vi "{TMPL} MAIN - App.vi"() -> ()   [LabVIEW 2015, in "TLB` Template.lvlib" / "{TMPL} TLB`.lvclass"]
uses:
  {TMPL} TLB`.lvclass
  Application Components/Trigger API/System Trigger.ctl
  State Machine/State.ctl
  Core Components/Error Handler/TLB` Error Handler.lvclass
  Application Components/Configuration/{TMPL} Station Configuration.lvclass
  {TMPL} TLB`.lvclass/{TMPL} TLB`.ctl
  <vilib>/Utility/error.llb/Error Cluster From Error Code.vi
  <vilib>/ErrorRing/Error Ring.xnode
  Application Components/Trigger API/{TMPL} Trigger API.lvlib
  TLB` Template.lvlib
  Core Components/Actions/Actions.lvlib
  Core Components/Dependencies/TLB`_Dependencies.lvlib
panel:
  out "error out":errorcluster
  out "State":string
  out "Status":string
  # "TLB` Template"
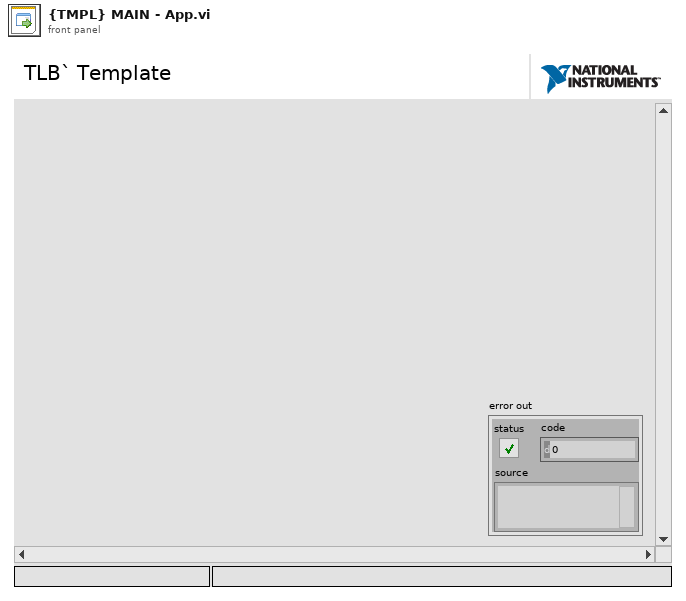
[diagram p1: front panel]
types:
  T1 = typedef "TLB` Template.lvlib/{TMPL} TLB`.lvclass/State.ctl" = enum16{"<Startup>", "Idle", "<Shutdown>", "<Error>"}
  T2 = enum16{"Close Display", "Clear References", "Close Error Handler"}
  T3 = enum16{"Clear SR", "Set Display", "Set Shifter", "Initialize Events", "Init Q"}
  T4 = typedef "TLB` Template.lvlib/{TMPL} Trigger API.lvlib/System Trigger.ctl" = enum16{"<None>", "Connect", "Start Acquisition", "Stop Acquisition", "Disconnect", "<Return to Safe State Actions>", "<Cache User Parameters>", "<Close Application>", "<Error>"}
  T5 = refnum<class "{TMPL} Station Configuration.lvclass">
  T6 = typedef "TLB` Template.lvlib/_UI CORE Event References.ctl" = cluster{"Exit Event":refnum<user-event>, "State Indicator":refnum<user-event>, "Status Indicator":refnum<user-event>}
  T7 = typedef "TLB` Template.lvlib/_UI APP Event References.ctl" = cluster{"Exit Event":refnum<user-event>}
  T8 = enum32{"Invalid", "Standard", "Closed", "Hidden", "Minimized", "Maximized"}
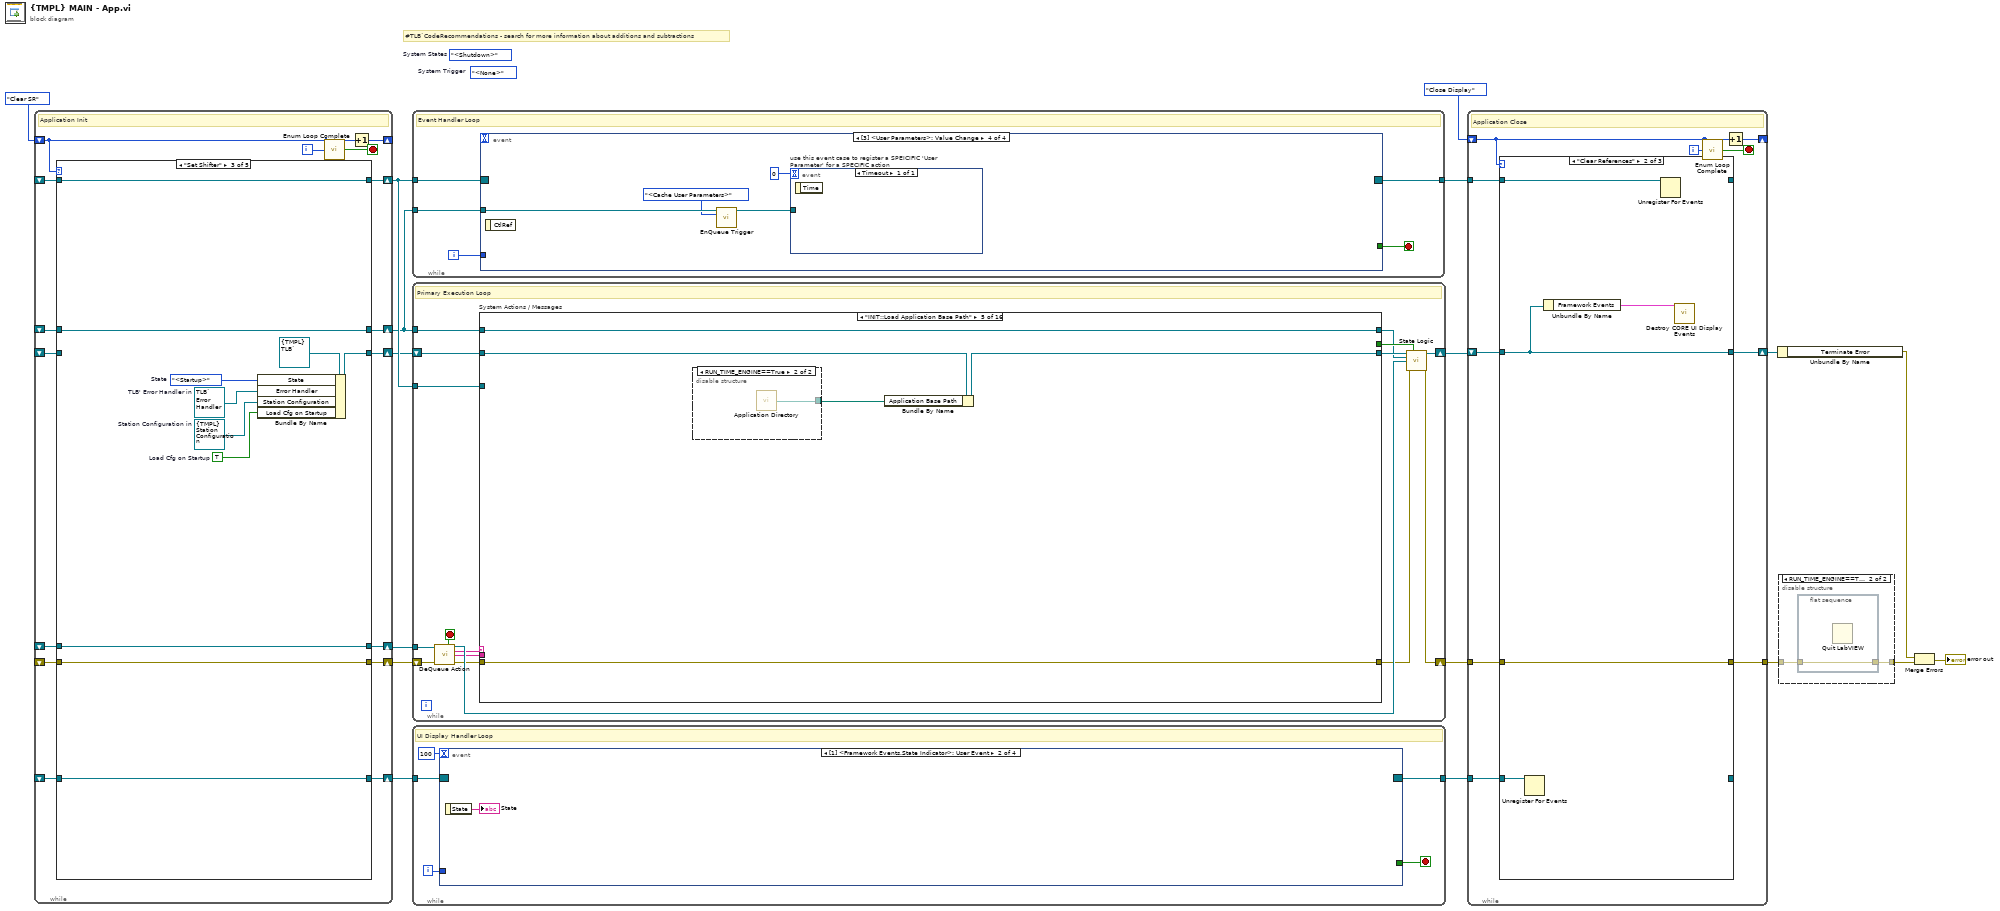
[diagram p0: block diagram]
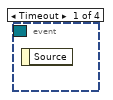
[diagram p2: hidden frame]
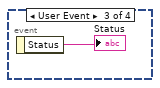
[diagram p3: hidden frame]
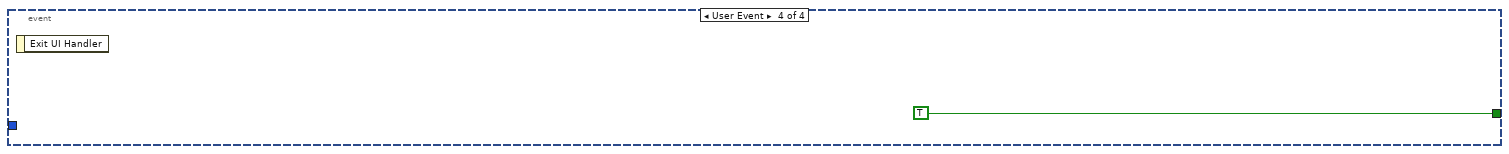
[diagram p4: hidden frame]
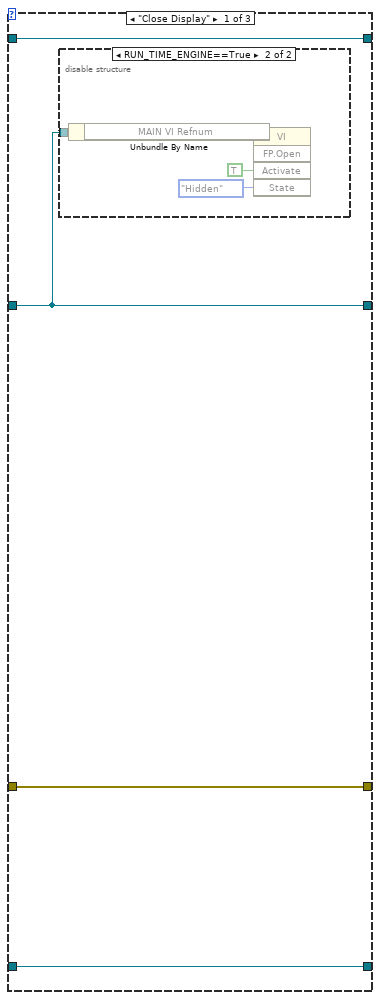
[diagram p6: hidden frame]
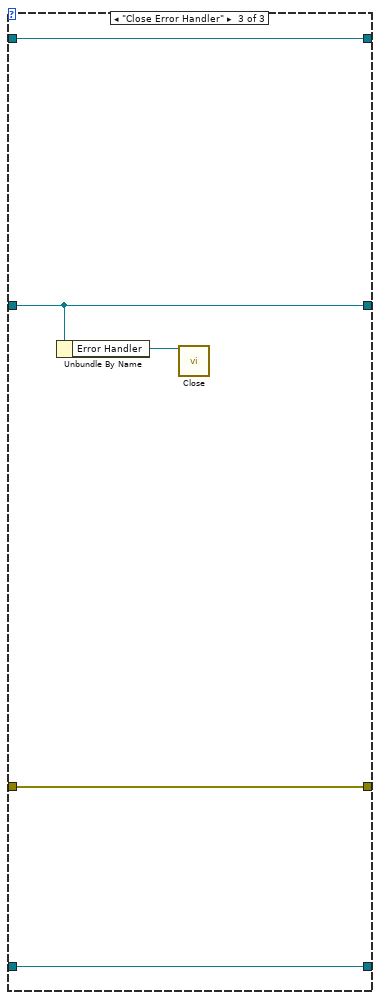
[diagram p8: hidden frame]
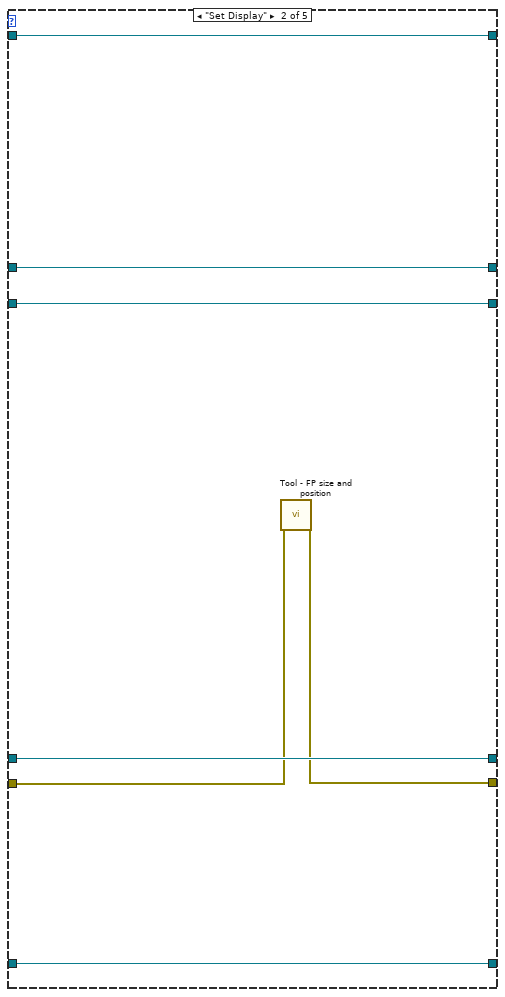
[diagram p10: hidden frame]
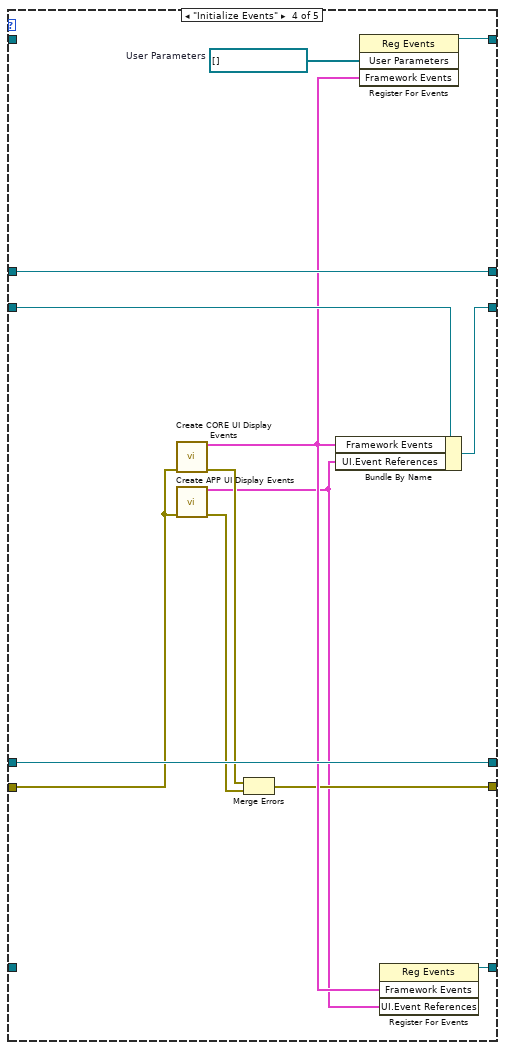
[diagram p11: hidden frame]
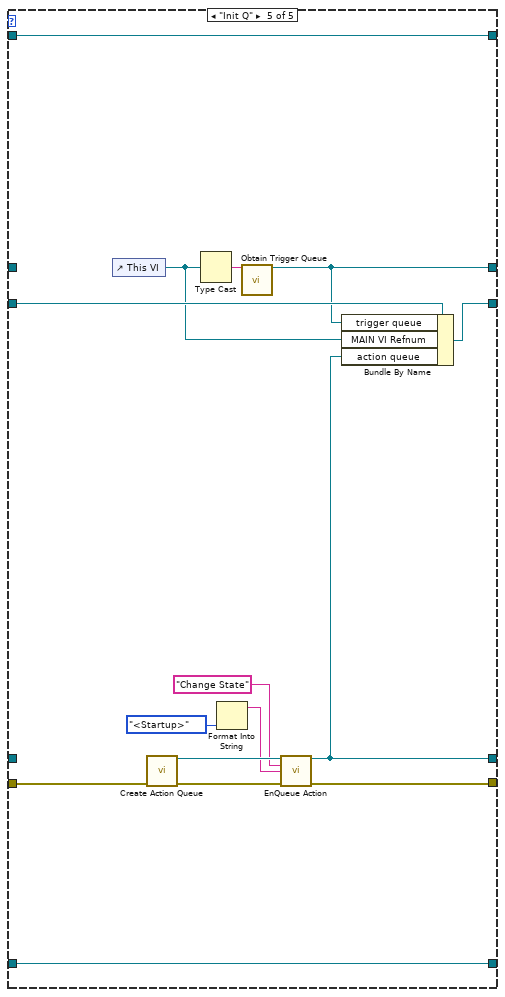
[diagram p12: hidden frame]
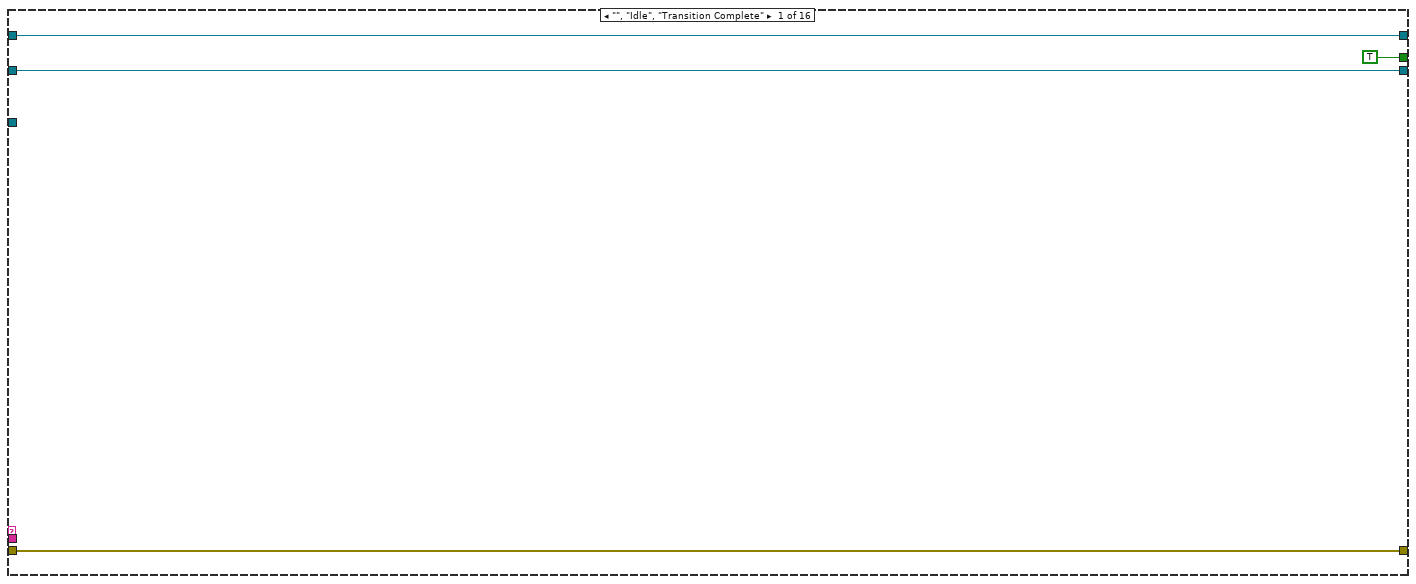
[diagram p13: hidden frame]
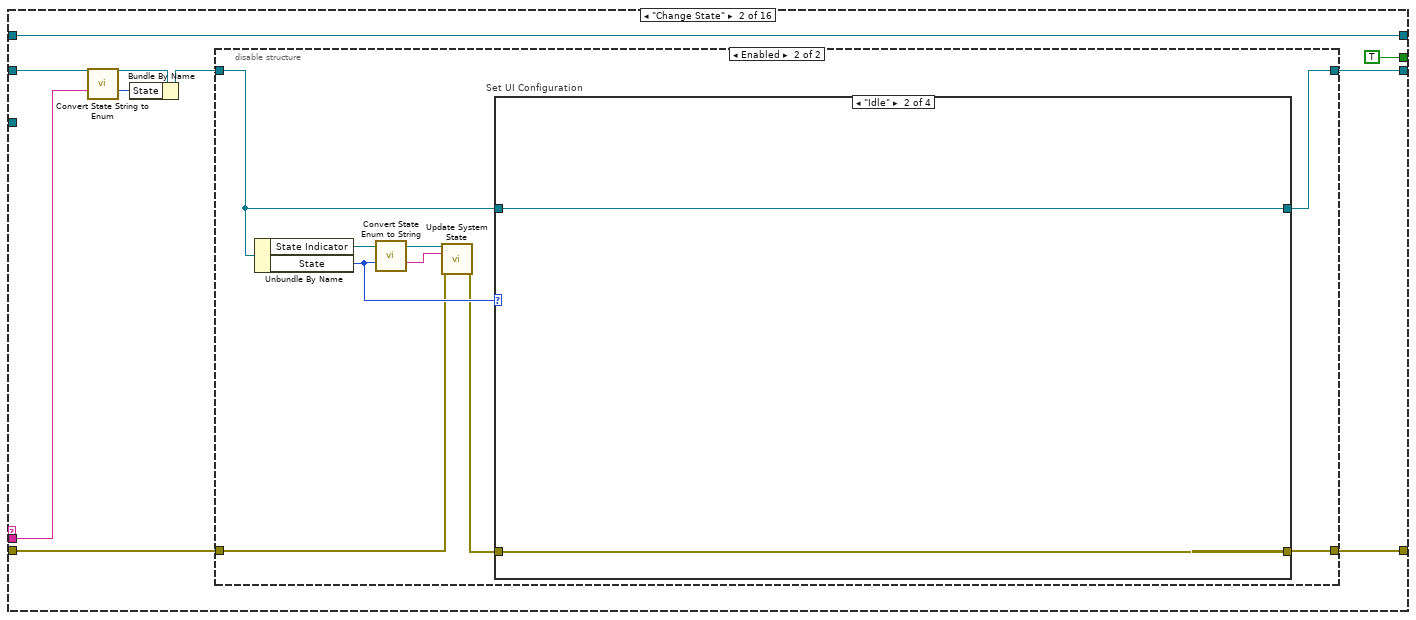
[diagram p14: hidden frame]
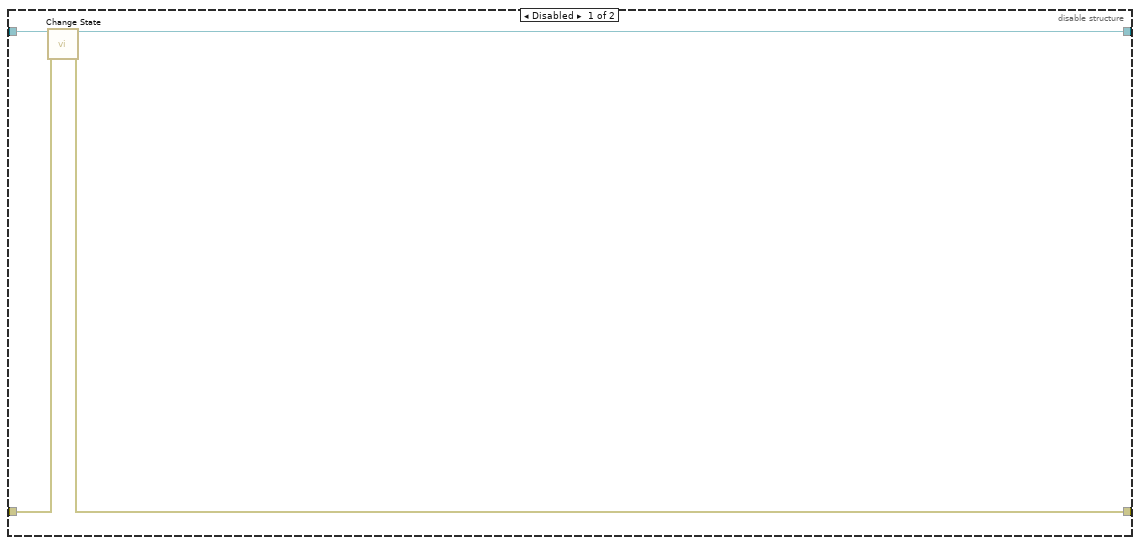
[diagram p15: hidden frame]
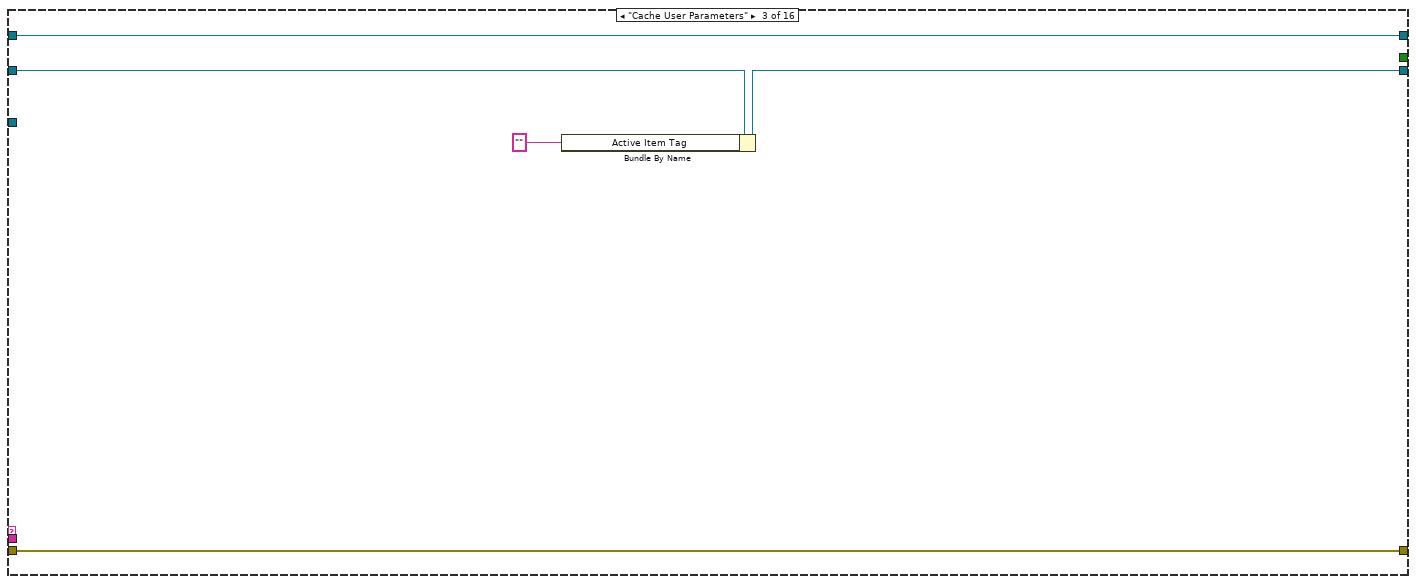
[diagram p19: hidden frame]
diagram:
  (unwired) State."<Shutdown>"  # System States
  (unwired) System_Trigger."<None>"  # System Trigger
  # "#TLB`CodeRecommendations - search for more information about additions and subtractions"
  n1 = while {
    shift-right: [w29] -> _
    shift-left: T3."Clear SR" -> [w18]
    shift-right: [w33] -> w17
    shift-left: _ -> [w28]
    shift-right: [w30] -> w12
    shift-left: _ -> [w27]
    shift-right: [w32] -> w11
    shift-left: _ -> [w26]
    shift-right: [w31] -> w10
    shift-left: _ -> [w25]
    shift-right: [w24] -> w6
    shift-left: _ -> [w23]
    shift-right: [w22] -> w9
    shift-left: _ -> [w21]
    i -> [w19]
    stop <- w20 stop-if-true
    # "Application Init"
    n2 = case shown="\"Set Shifter\"" w18 {
      tunnel: [_ w38 w51 w64 w65] -> w33
      tunnel: [_ w36 w50 w54 w71] -> w30
      tunnel: [_ w40 w46 w62 w77] -> w31
      tunnel: [_ w39 w49 w61 w79] -> w32
      tunnel: w28 -> [_ w38 w51 w64 _]
      tunnel: w27 -> [_ w37 w50 w53 w73]
      tunnel: w26 -> [_ w39 w49 _ w79]
      tunnel: w25 -> [_ w40 _ w63 w78]
      tunnel: [_ w35 w48 w60 w66] -> w24
      tunnel: w23 -> [_ w35 w48 w60 _]
      tunnel: [_ w34 w44 w58 w74] -> w22
      tunnel: w21 -> [_ w34 w44 _ w74]
      frame "Clear SR" {
      }
      frame "Set Display" {
        n3 = call "Tool - FP size and position.vi"("error in (no error)"=w37) -> ("error out"=w36:errorcluster)  [unwired: 17 in, 1 out]
      }
      frame "Set Shifter" {
        w41 = TRUE  # Load Cfg on Startup
        w42 = T5 refnum  # Station Configuration in
        w43 = refnum<class "TLB` Error Handler.lvclass"> refnum  # TLB' Error Handler in
        w47 = State."<Startup>"  # State
        n4 = Bundle By Name(cluster=refnum<class "{TMPL} TLB`.lvclass"> refnum ("TLB` Template.lvlib:TLB' Template.lvclass"), "State"=w47, "Error Handler"=w43, "Station Configuration"=w42, "Load Cfg on Startup"=w41) -> (w46:refnum<class "{TMPL} TLB`.lvclass">)
      }
      frame "Initialize Events" {
        w59 = refnum<vi>[] []  # User Parameters
        n5 = call "Create CORE UI Display Events.vi"("error in"=w53) -> ("Framework Events"=w57:T6, "error out"=w56:errorcluster)  [unwired: 13 in]
        n6 = call "Create APP UI Display Events.vi"("error in"=w53) -> ("UI.Event References"=w52:T7, "error out"=w55:errorcluster)  [unwired: 13 in]
        n7 = Merge Errors(w56, w55) -> (w54:errorcluster)
        n8 = Bundle By Name(cluster=w63, "Framework Events"=w57, "UI.Event References"=w52) -> (w62:refnum<class "{TMPL} TLB`.lvclass">)
        n9 = register-events(w59, w57) -> (reference out=w61:refnum<event-registration>)  [unwired: 2 in, 1 out]
        n10 = register-events(w57, w52) -> (reference out=w58:refnum<event-registration>)  [unwired: 2 in, 1 out]
      }
      frame "Init Q" {
        n11 = control-ref of="This VI"() -> (w76:refnum<vi>)
        n12 = call "Create Action Queue.vi"("error in"=w73) -> ("action queue out"=w70:refnum<queue>, "error out"=w72:errorcluster)  [unwired: 13 in]
        n13 = Type Cast(x=w76) -> (*(type *) &x=w67:string)  [unwired: 1 in]
        n14 = Format Into String(State."<Startup>" ("State")) -> (resulting string=w68:string)  [unwired: 3 in, 1 out]
        n15 = call "Obtain Trigger Queue.vi"("trigger queue name"=w67) -> ("trigger queue out"=w66:refnum<queue>)  [unwired: 13 in, 1 out]
        n16 = call "EnQueue Action.vi"("action queue in"=w70, "action"="Change State" ("Message Name"), "data in"=w68, "error in"=w72) -> ("action queue out"=w65:refnum<queue>, "error out"=w71:errorcluster)  [unwired: 10 in]
        n17 = Bundle By Name(cluster=w78, "trigger queue"=w66, "MAIN VI Refnum"=w76, "action queue"=w65) -> (w77:refnum<class "{TMPL} TLB`.lvclass">)
      }
    }
    n18 = call "Enum Loop Complete.vi"("Current State Enum"=w18, "Itteration"=w19) -> ("Loop Complete?"=w20:bool)  [unwired: 12 in, 1 out]
    n19 = Increment(x=w18) -> (x+1=w29:T3)
  }
  n20 = while {
    shift-right: [w90] -> w8
    shift-left: w12 -> [w85]
    shift-right: [w92] -> w13
    shift-left: w10 -> [w94]
    tunnel: w17 -> [w86]
    tunnel: w11 -> [w93]
    tunnel: w6 -> [w89]
    stop <- w84 stop-if-true
    # "Primary Execution Loop"
    n21 = call "DeQueue Action.vi"("action queue in"=w86, "error in"=w85) -> ("exit?"=w84:bool, "action queue out"=w95:refnum<queue>, "action"=w82:string, "action value"=w80:string, "error out"=w83:errorcluster)  [unwired: 8 in, 1 out]
    n22 = case "System Actions / Messages" shown="\"INIT::Load Application Base Path\"" w82 {
      selector: w82 -> [_ _ _ _ _ _ _ _ _ _ _ _ _ _ _ w225]
      tunnel: [w99 w106 w132 w136 w137 w145 w162 w174 w177 w184 w197 w202 w207 w208 w220 w224] -> w87
      tunnel: w83 -> [w99 w105 w132 w136 w137 w148 w162 w174 w177 w182 w197 w201 w207 w209 w221 _]
      tunnel: w94 -> [w96 w104 w129 w135 w140 w146 w165 w173 w176 w181 w196 w204 w206 w212 w223 w227]
      tunnel: [w96 w100 w133 w135 w139 w151 w168 w173 w176 w178 w196 w204 w206 w211 w222 w227] -> w91
      tunnel: w93 -> [_ _ _ _ _ _ w166 _ _ _ _ _ _ _ _ _]
      tunnel: [w97 w107 w131 w134 w141 w152 w167 w172 w175 w187 w195 w199 w205 w215 w216 w226] -> w81
      tunnel: w89 -> [w97 w107 w131 w134 w141 w152 w167 w172 w175 w187 w195 w199 w205 w215 w216 w226]
      tunnel: [TRUE TRUE _ _ _ _ _ _ _ _ _ _ _ _ _ _] -> w88
      tunnel: w80 -> [_ w103 _ _ _ _ _ _ _ _ _ _ _ _ _ _]
      frame "", "Idle", "Transition Complete" {
      }
      frame "Change State" {
        n23 = call "Convert State String to Enum.vi"("state in"=w103) -> ("state out"=w102:T1)  [unwired: 13 in, 1 out]
        n24 = Bundle By Name(cluster=w104, "State"=w102) -> (w101:refnum<class "{TMPL} TLB`.lvclass">)
        n25 = disable-structure shown="Enabled" {
          disable-tunnel: [w112 w113] -> w106
          disable-tunnel: w105 -> [w111 w114]
          disable-tunnel: w101 -> [w110 w116]
          disable-tunnel: [w109 w115] -> w100
          frame Disabled {
            n26 = call "Change State.vi"("TLB' data in"=w110, "error in"=w111) -> ("TLB' data out"=w109:refnum<class "{TMPL} TLB`.lvclass">, "error out"=w112:errorcluster)  [unwired: 12 in]
          }
          frame Enabled {
            n27 = Unbundle By Name(w116) -> ("State Indicator"=w117:refnum<user-event>, "State"=w120:T1)
            n28 = call "Convert State Enum to String.vi"("state in"=w120) -> ("state out"=w118:string)  [unwired: 13 in, 1 out]
            n29 = call "Update System State.vi"("State Indicator"=w117, "system state message"=w118, "error in"=w114) -> ("error out"=w119:errorcluster)  [unwired: 12 in]
            n30 = case "Set UI Configuration" shown="\"Idle\"" w120 {
              tunnel: [w121 w124 w125 w128] -> w113
              tunnel: w119 -> [w121 w124 w125 w128]
              tunnel: [w122 w123 w126 w127] -> w115
              tunnel: w116 -> [w122 w123 w126 w127]
              frame "<Startup>" {
              }
              frame "Idle" {
              }
              frame "<Error>" {
              }
              frame "<Shutdown>" {
              }
            }
          }
        }
      }
      frame "Cache User Parameters" {
        n31 = Bundle By Name(cluster=w129, "Active Item Tag"="" ("User Data.Active Item Tag")) -> (w133:refnum<class "{TMPL} TLB`.lvclass">)
      }
      frame "/*********INITialize********/" {
      }
      frame "INIT::Load Application Base Path" {
        n32 = disable-structure shown="RUN_TIME_ENGINE==True" {
          disable-tunnel: [w142 w144] -> w138
          frame condition #0 (active) {
            n33 = Current VI's Path() -> (path=w143:path)
            n34 = Strip Path(path=w143) -> (stripped path=w142:path)  [unwired: 1 out]
          }
          frame condition #1 {
            n35 = call <vilib>:"Application Directory.vi"() -> ("Application Directory"=w144:path)
          }
        }
        n36 = Bundle By Name(cluster=w140, "Application Base Path"=w138) -> (w139:refnum<class "{TMPL} TLB`.lvclass">)
      }
      frame "INIT::Initialize Error Handler" {
        n37 = disable-structure shown="Default" {
          disable-tunnel: [w156 w159] -> w153
          disable-tunnel: ["System Level Errors\\System Errors.txt" ("name or relative path") "System Level Errors\\System Errors.txt" ("name or relative path")] -> w154
          disable-tunnel: w146 -> [w155 w161]
          frame condition #0 (active) {
            n38 = Unbundle By Name(w155) -> ("Application Base Path"=w156:path)
          }
          frame condition #1 {
            n39 = Unbundle By Name(w161) -> ("Application Base Path"=w160:path)
            n40 = Strip Path(path=w160) -> (stripped path=w159:path)  [unwired: 1 out]
          }
        }
        n41 = Unbundle By Name(w146) -> ("Error Handler"=w147:refnum<class "TLB` Error Handler.lvclass">)
        n42 = Build Path(base path=w153, name or relative path=w154) -> (appended path=w149:path)
        n43 = call-dynamic "Open.vi"("error handler in"=w147, "error log path in"=w149, "error in"=w148) -> ("error handler out"=w150:refnum<class "TLB` Error Handler.lvclass">, "error out"=w145:errorcluster)  [unwired: 11 in]
        n44 = Bundle By Name(cluster=w146, "Error Handler"=w150) -> (w151:refnum<class "{TMPL} TLB`.lvclass">)
      }
      frame "INIT::Register User Parameters" {
        n45 = disable-structure shown="Disabled" {
          disable-tunnel: [w169 refnum<vi>[] [] ("User Parameter Controls")] -> w164
          frame Disabled {
            n46 = stacked-sequence "Stacked Sequence Structure :: Allows for a lot of controls" {
              tunnel: [w170] -> w169
              frame #0 {
                n47 = Build Array() -> (w170:void[])  [unwired: 4 in]
              }
            }
          }
          frame Enabled {
          }
        }
        n48 = Build Array (concatenate)(w164) -> (w163:refnum<vi>[])
        n49 = register-events(reference=w166, w163) -> ()  [unwired: 2 in, 2 out]
        n50 = Bundle By Name(cluster=w165, "User Parameter Controls"=w163) -> (w168:refnum<class "{TMPL} TLB`.lvclass">)
      }
      frame "INIT::FP Values" {
        # "#TLB`CodeRecommendations - initialize FP values here"
      }
      frame "/*********PRImary EXEcution********/" {
      }
      frame "CFG::Load Station Configuration" {
        n51 = disable-structure shown="RUN_TIME_ENGINE==True" {
          disable-tunnel: [w189 w192] -> w186
          disable-tunnel: ["System Configuration\\Station Configuration.ini" ("name or relative path") "System Configuration\\Station Configuration.ini" ("name or relative path")] -> w185
          disable-tunnel: w181 -> [w188 w193]
          frame condition #0 (active) {
            n52 = Unbundle By Name(w188) -> ("Application Base Path"=w189:path)
          }
          frame condition #1 {
            n53 = Unbundle By Name(w193) -> ("Application Base Path"=w194:path)
            n54 = Strip Path(path=w194) -> (stripped path=w192:path)  [unwired: 1 out]
          }
        }
        n55 = Unbundle By Name(w181) -> ("Station Configuration"=w180:T5)
        n56 = Build Path(base path=w186, name or relative path=w185) -> (appended path=w183:path)
        n57 = call-dynamic "Load Configuration.vi"("INI Station Configuration in"=w180, "INI file path in"=w183, "error in"=w182) -> ("INI Station Configuration out"=w179:T5, "error out"=w184:errorcluster)  [unwired: 11 in]
        n58 = Bundle By Name(cluster=w181, "Station Configuration"=w179) -> (w178:refnum<class "{TMPL} TLB`.lvclass">)
      }
      frame "/*********SHUTDOWN********/" {
      }
      frame "Exit" {
        w200 = refnum<class> refnum  # event data
        # "Don't wire 'Error In'\nMust Execute Regardless"
        n59 = Unbundle By Name(w204) -> ("Exit Event"=w198:refnum<user-event>)
        n60 = Generate User Event(user event=w198, event data cluster=w200) -> (error out=w203:errorcluster)  [unwired: 2 in, 1 out]
        n61 = Merge Errors(w201, w203) -> (w202:errorcluster)
      }
      frame "/*********ERRor Handler********/" {
      }
      frame "ERR::Log" {
        n62 = Unbundle By Name(w212) -> ("Error Handler"=w214:refnum<class "TLB` Error Handler.lvclass">)
        n63 = call-dynamic "Log.vi"("error handler in"=w214) -> ("error handler out"=w213:refnum<class "TLB` Error Handler.lvclass">, "error out"=w210:errorcluster)  [unwired: 13 in]
        n64 = Bundle By Name(cluster=w212, "Error Handler"=w213) -> (w211:refnum<class "{TMPL} TLB`.lvclass">)
        n65 = Merge Errors(w209, w210) -> (w208:errorcluster)
      }
      frame "ERR::Dialog" {
        n66 = Unbundle By Name(w223) -> ("Error Handler"=w219:refnum<class "TLB` Error Handler.lvclass">)
        n67 = call-dynamic "Dialog.vi"("error handler in"=w219, "trigger queue in"=w216) -> ("error handler out"=w218:refnum<class "TLB` Error Handler.lvclass">, "error out"=w217:errorcluster)  [unwired: 12 in]
        n68 = Merge Errors(w221, w217) -> (w220:errorcluster)
        n69 = Bundle By Name(cluster=w223, "Error Handler"=w218) -> (w222:refnum<class "{TMPL} TLB`.lvclass">)
      }
      frame Default {
        n70 = xnode "Error Ring"("parameter 0"=w225) -> ("error out"=w224:errorcluster)
      }
    }
    n71 = call "State Logic.vi"("TLB' data in"=w91, "process state logic enable"=w88, "trigger queue in"=w81, "action queue in"=w95, "error in"=w87) -> ("TLB' data out"=w92:refnum<class "{TMPL} TLB`.lvclass">, "error out"=w90:errorcluster)  [unwired: 9 in]
  }
  n72 = while {
    tunnel: w9 -> [w239]
    tunnel: [w235] -> w7
    i -> [w238]
    stop <- w237 stop-if-true
    # "UI Display Handler Loop"
    n73 = event shown="[1] <Framework Events.State Indicator>: User Event" {
      selector: w239 -> [_ _ _ _]
      dyn-events: [_ _ _ _] -> w235
      timeout: 100 -> [_ _ _ _]
      tunnel: w238 -> [_ _ _ _]
      tunnel: [_ _ _ TRUE] -> w237
      event Timeout {
        n74 = event-data() -> ()  [unwired: 2 out]
      }
      event User Event {
        n75 = event-data() -> ("State"=→"State":string)  [unwired: 1 out]
      }
      event User Event {
        n76 = event-data() -> ("Status"=→"Status":string)  [unwired: 1 out]
      }
      event User Event {
        n77 = event-data() -> ()  [unwired: 2 out]
      }
    }
  }
  n78 = while {
    tunnel: w11 -> [w246]
    tunnel: [w245] -> w14
    tunnel: w6 -> [w243]
    i -> [w244]
    stop <- w247 stop-if-true
    # "Event Handler Loop"
    n79 = event shown="[3] <User Parameters>: Value Change" {
      selector: w246 -> [_ _ _ _]
      dyn-events: [_ _ _ _] -> w245
      timeout: _ -> [_ _ _ _]
      tunnel: [_ _ TRUE ("NewVal") _] -> w247
      tunnel: w244 -> [_ _ _ _]
      tunnel: w243 -> [w248 _ w260 w264]
      event Panel Close? {
        w250 = TRUE  # Discard?
        n80 = event-data() -> ()  [unwired: 2 out]
        n81 = call "EnQueue Trigger.vi"("trigger queue in"=w248, "system trigger"=System_Trigger."<Close Application>" ("System Trigger")) -> ()  [unwired: 12 in, 2 out]
        n82 = event-data("Discard?"=w250) -> ()  [unwired: 1 in, 1 out]
      }
      event Mouse Down {
        n83 = event-data() -> ("Button"=w251:u16, "Mods.Double Click"=w252:bool)  [unwired: 1 out]
        n84 = Equal?(x=u16 2, y=w251) -> (x = y?=w254:bool)
        n85 = Compound Arithmetic op=AND(w254, w252) -> (w253:bool)
        n86 = case "Toggle Menu Visibility :: double RIGHT click on logo" shown="True" w253 {
          frame False {
          }
          frame True {
            n87 = property class="VI"() -> (reference out=w258:refnum<vi>, "TB.Visible"=w256:bool)  [unwired: 2 in, 1 out]
            n88 = Not(x=w256) -> (.not. x?=w257:bool)
            n89 = property class="VI"(reference=w258, "TB.Visible"=w257) -> ()  [unwired: 1 in, 2 out]
          }
        }
      }
      event User Event {
        n90 = event-data() -> ()  [unwired: 2 out]
        n91 = call "EnQueue Trigger.vi"("trigger queue in"=w260, "system trigger"=System_Trigger."<Close Application>" ("System Trigger")) -> ()  [unwired: 12 in, 2 out]
      }
      event Value Change {
        n92 = event-data() -> ()  [unwired: 2 out]
        n93 = call "EnQueue Trigger.vi"("trigger queue in"=w264, "system trigger"=System_Trigger."<Cache User Parameters>" ("System Trigger")) -> ("trigger queue out"=w263:refnum<queue>)  [unwired: 12 in, 1 out]
        n94 = event "use this event case to register a SPEICIFIC 'User Parameter' for a SPECIFIC action" shown="[0] Timeout" {
          selector: _ -> [_]
          dyn-events: _ -> [_]
          timeout: 0 -> [_]
          tunnel: w263 -> [_]
          event Timeout {
            n95 = event-data() -> ()  [unwired: 1 in, 1 out]
          }
        }
      }
    }
  }
  n96 = while {
    shift-right: [w275] -> _
    shift-left: T2."Close Display" -> [w268]
    tunnel: w14 -> [w273]
    tunnel: w8 -> [w274]
    tunnel: [w271] -> w16
    shift-right: [w270] -> w4
    shift-left: w13 -> [w272]
    tunnel: w7 -> [w269]
    i -> [w266]
    stop <- w267 stop-if-true
    # "Application Close"
    n97 = case shown="\"Clear References\"" w268 {
      tunnel: [w278 w288 w293] -> w271
      tunnel: [w277 w287 w290] -> w270
      tunnel: [w279 _ w292] -> _
      tunnel: w274 -> [w278 w288 w293]
      tunnel: w273 -> [w279 w286 w292]
      tunnel: w272 -> [w277 w287 w290]
      tunnel: w269 -> [w276 w284 w291]
      tunnel: [w276 _ w291] -> _
      frame "Close Display" {
        n98 = disable-structure shown="RUN_TIME_ENGINE==True" {
          disable-tunnel: w277 -> [_ w281]
          frame condition #0 (active) {
          }
          frame condition #1 {
            n99 = Unbundle By Name(w281) -> ("MAIN VI Refnum"=w280:refnum<vi>)
            n100 = invoke class="VI" method="FP.Open"(reference=w280, "Activate"=TRUE ("Activate?"), "State"=T8."Hidden") -> ()  [unwired: 2 in, 5 out]
          }
        }
      }
      frame "Clear References" {
        n101 = Unregister For Events(event registration refnum=w284) -> ()  [unwired: 1 in, 1 out]
        n102 = Unbundle By Name(w287) -> ("Framework Events"=w285:T6)
        n103 = Unregister For Events(event registration refnum=w286) -> ()  [unwired: 1 in, 1 out]
        n104 = call "Destroy CORE UI Display Events.vi"("UI display events in"=w285) -> ()  [unwired: 14 in, 1 out]
      }
      frame "Close Error Handler" {
        n105 = Unbundle By Name(w290) -> ("Error Handler"=w289:refnum<class "TLB` Error Handler.lvclass">)
        n106 = call-dynamic "Close.vi"("error handler in"=w289) -> ()  [unwired: 14 in, 1 out]
      }
    }
    n107 = call "Enum Loop Complete.vi"("Current State Enum"=w268, "Itteration"=w266) -> ("Loop Complete?"=w267:bool)  [unwired: 12 in, 1 out]
    n108 = Increment(x=w268) -> (x+1=w275:T2)
  }
  n109 = Unbundle By Name(w4) -> ("Terminate Error"=w3:errorcluster)
  n110 = disable-structure shown="RUN_TIME_ENGINE==True" {
    disable-tunnel: [w294 w295] -> w2
    disable-tunnel: w16 -> [w294 w296]
    frame condition #0 (active) {
    }
    frame condition #1 {
      n111 = flat-sequence {
        tunnel: [w297] -> w295
        tunnel: w296 -> [w297]
        frame #0 {
          n112 = Quit LabVIEW() -> ()  [unwired: 1 in]
        }
      }
    }
  }
  n113 = Merge Errors(w3, w2) -> (→"error out":errorcluster)
